vi "Buttons and color.vi"() -> ()   [LabVIEW 2025]
panel:
  in  "Folding":bool
  in  "Configuration":bool
  out "Time":dbl format="%<%H:%M:%S>t"
  in  "Start Test 5":bool
  in  "Start Test 4":bool
  in  "Start Test 3":bool
  in  "Remote":bool
  in  "Minimize":bool
  in  "Maximize":bool
  in  "Close":bool
  out "Start 2":bool
  in  "Start":bool
  in  "Start Test 2":bool
  in  "Stop":bool
  in  "Account 4":bool
  in  "Account 3":bool
  in  "Save Menu":u16(ring)
  in  "Open":bool
  in  "New":bool
  in  "Account":bool
  in  "View Sequence":bool
  in  "Settings":bool
  # "118,199,124"
  # "0,172,217"
  # "186,12,47"
  # "255,215,0"
  # "99,102.106"
  # "167,168,170"
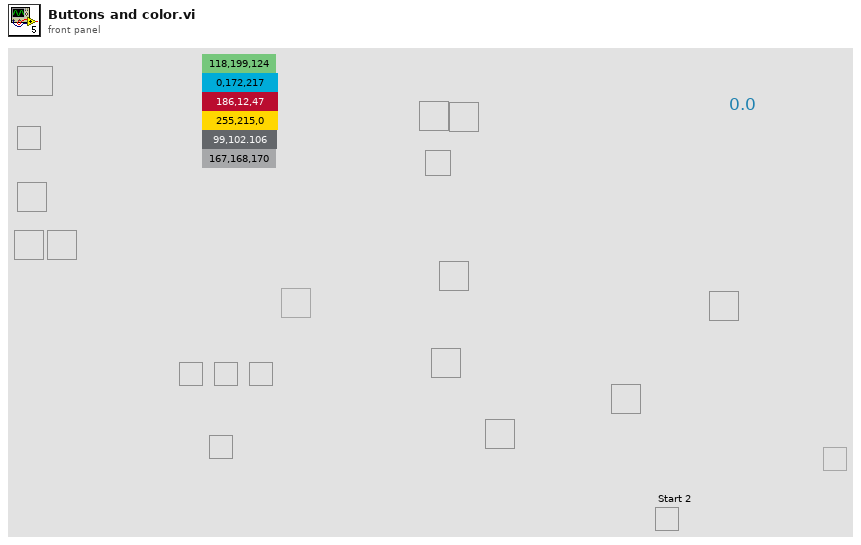
[diagram p1: front panel]
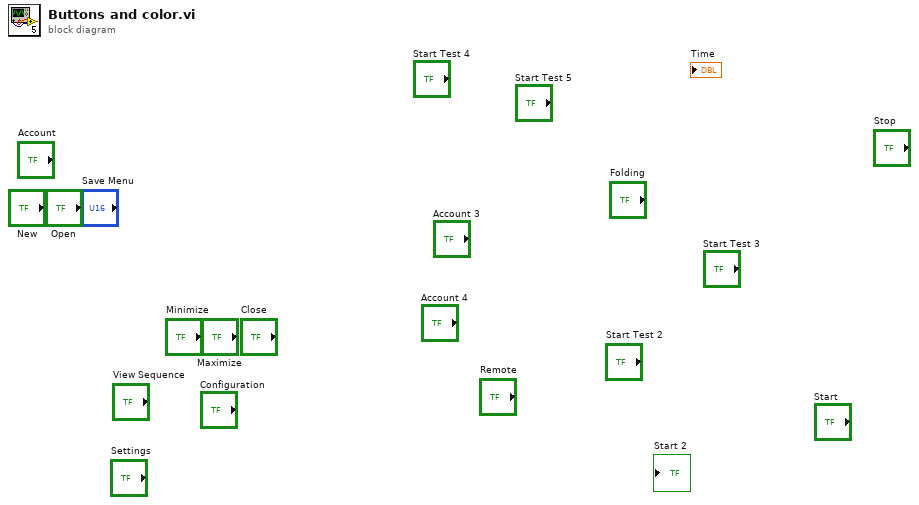
[diagram p0: block diagram]
diagram:
